vi "08 - Tip - Achieving Deterministic Handling Order.vi"() -> ()   [LabVIEW 2012]
panel:
  in  "Generate Events":enum16{"Greater than 1msec", "Sub-millisecond"}(ring)
  in  "Control":bool
  out "Static Event Registration":i32(graph)
  out "Dynamic Event Registration":i32(graph)
  out "Unique Event Queue":i32(graph)
  # "Conclusion:\nAll events within a single Events Queue will be handled deterministically;\nevents in separate Events Queues will be handled with approximately millisecond\naccuracy, but could become out of order with sub-millisecond resolution.\n\nNever expect deterministic handling order between separate event registrations,\nbut especially near and below 1msec threshold."
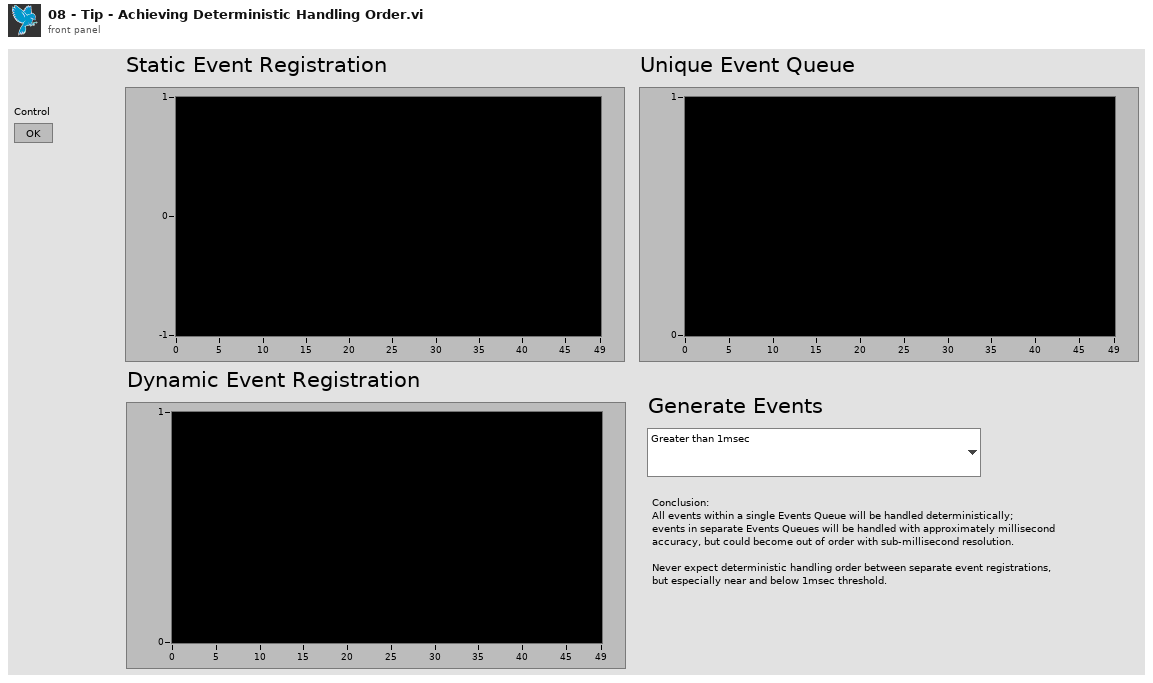
[diagram p1: front panel]
types:
  T1 = cluster{"Event Registration Refnum":refnum<event-registration>, "Event Registration Refnum":refnum<event-registration>}
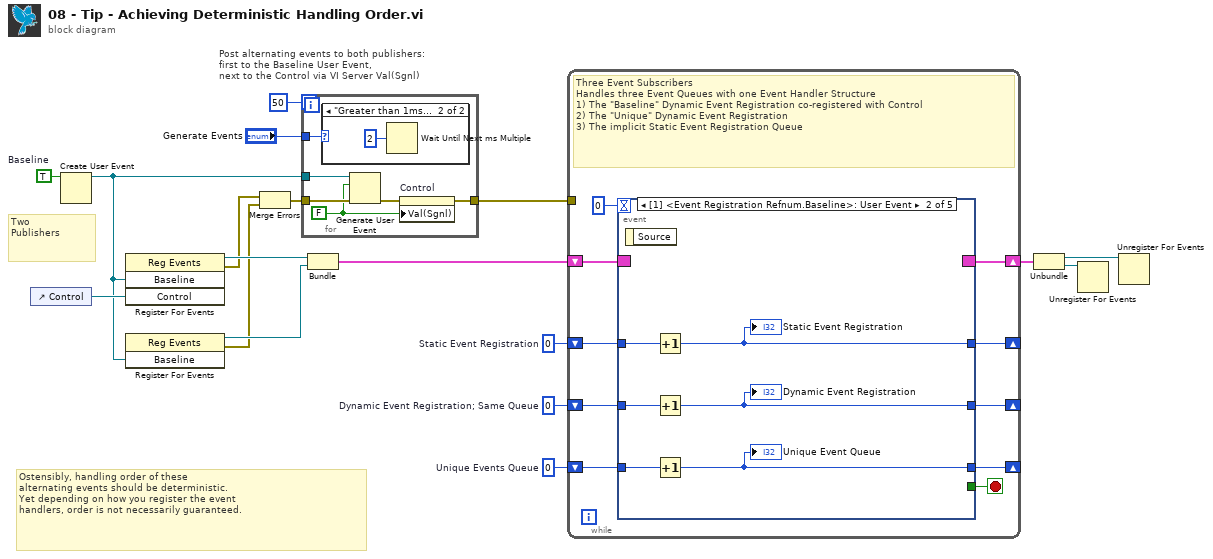
[diagram p0: block diagram]
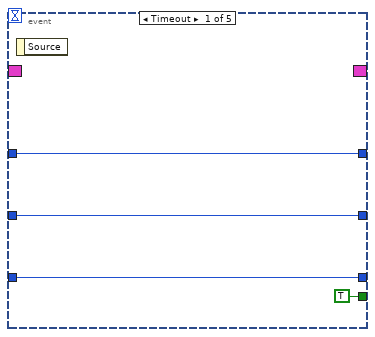
[diagram p3: hidden frame]
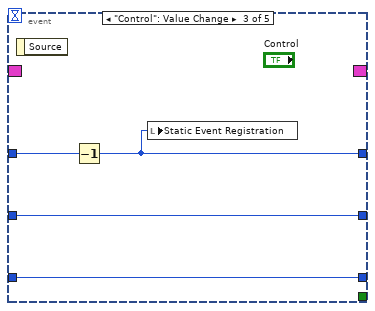
[diagram p4: hidden frame]
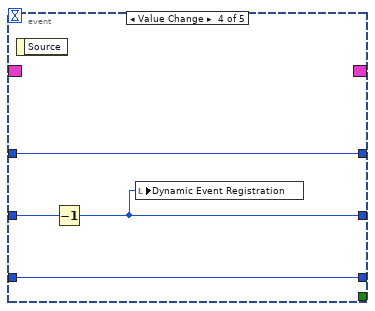
[diagram p5: hidden frame]
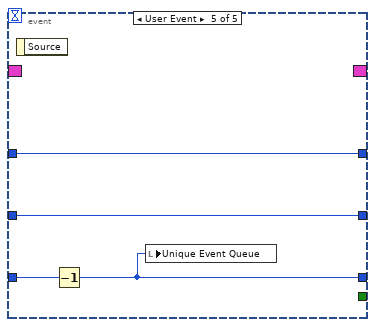
[diagram p6: hidden frame]
diagram:
  w8 = 0  # Unique Events Queue
  w13 = 0  # Dynamic Event Registration; Same Queue
  w15 = 0  # Static Event Registration
  w18 = TRUE  # Baseline
  # "Two\nPublishers"
  # "Ostensibly, handling order of these\nalternating events should be deterministic.\nYet depending on how you register the event\nhandlers, order is not necessarily guaranteed."
  n1 = control-ref of="Control"() -> (w14:refnum<vi>)
  n2 = Create User Event(user event datatype=w18) -> (user event=w12:refnum<user-event>)  [unwired: 1 in, 1 out]
  n3 = register-events(w12, w14) -> (reference out=w11:refnum<event-registration>, error out=w7:errorcluster)  [unwired: 2 in]
  n4 = register-events(w12) -> (reference out=w9:refnum<event-registration>, error out=w6:errorcluster)  [unwired: 2 in]
  n5 = Merge Errors(w7, w6) -> (w5:errorcluster)
  n6 = for "Post alternating events to both publishers:\nfirst to the Baseline User Event,\nnext to the Control via VI Server Val(Sgnl)" {
    N: 50 -> [_]
    tunnel: w12 -> [w23]
    tunnel: w5 -> [w22]
    tunnel: [w21] -> w16
    tunnel: "Generate Events" -> [w19]
    w20 = FALSE ("Value (Signaling)")
    n7 = case shown="\"Greater than 1msec\"" w19 {
      frame "Sub-millisecond" {
      }
      frame "Greater than 1msec" {
        n8 = Wait Until Next ms Multiple(millisecond multiple=u32 2 ("milliseconds to wait")) -> ()  [unwired: 1 out]
      }
    }
    n9 = Generate User Event(user event=w23, event data cluster=w20, error in=w22) -> (error out=w24:errorcluster)  [unwired: 1 out]
    n10 = property on="Control" class="Bool (strict)"(error in=w24, "Val(Sgnl)"=w20) -> (error out=w21:errorcluster)  [unwired: 1 in, 1 out]
  }
  n11 = Bundle("Event Registration Refnum"=w11, "Event Registration Refnum"=w9) -> (w10:T1)  [unwired: 1 in]
  n12 = while {
    tunnel: w16 -> [_]
    shift-right: [w31] -> _
    shift-left: w15 -> [w32]
    shift-right: [w29] -> _
    shift-left: w13 -> [w30]
    shift-right: [w28] -> _
    shift-left: w8 -> [w27]
    shift-right: [w26] -> w3
    shift-left: w10 -> [w35]
    stop <- w34 stop-if-true
    # "Three Event Subscribers\nHandles three Event Queues with one Event Handler Structure\n1) The \"Baseline\" Dynamic Event Registration co-registered with Control\n2) The \"Unique\" Dynamic Event Registration\n3) The implicit Static Event Registration Queue"
    n13 = event shown="[1] <Event Registration Refnum.Baseline>: User Event" {
      selector: w35 -> [_ _ _ _ _]
      dyn-events: [_ _ _ _ _] -> w26
      timeout: 0 -> [_ _ _ _ _]
      tunnel: [TRUE _ _ _ _] -> w34
      tunnel: w32 -> [w38 w45 w49 w52 w57]
      tunnel: [w38 w40 w46 w52 w57] -> w31
      tunnel: w30 -> [w37 w44 w48 w53 w55]
      tunnel: [w37 w41 w48 w50 w55] -> w29
      tunnel: [w36 w42 w47 w51 w54] -> w28
      tunnel: w27 -> [w36 w43 w47 w51 w56]
      event Timeout {
        n14 = event-data() -> ()  [unwired: 1 in, 1 out]
      }
      event User Event {
        n15 = event-data() -> ()  [unwired: 1 in, 1 out]
        n16 = Increment(x=w45) -> (x+1=w40:i32)
        "Static Event Registration" <- w40
        n17 = Increment(x=w44) -> (x+1=w41:i32)
        "Dynamic Event Registration" <- w41
        n18 = Increment(x=w43) -> (x+1=w42:i32)
        "Unique Event Queue" <- w42
      }
      event "Control": Value Change {
        n19 = event-data() -> ()  [unwired: 1 in, 1 out]
        n20 = Decrement(x=w49) -> (x-1=w46:i32)
        n21 = local write "Static Event Registration"(w46) -> ()
      }
      event Value Change {
        n22 = event-data() -> ()  [unwired: 1 in, 1 out]
        n23 = Decrement(x=w53) -> (x-1=w50:i32)
        n24 = local write "Dynamic Event Registration"(w50) -> ()
      }
      event User Event {
        n25 = event-data() -> ()  [unwired: 1 in, 1 out]
        n26 = Decrement(x=w56) -> (x-1=w54:i32)
        n27 = local write "Unique Event Queue"(w54) -> ()
      }
    }
  }
  n28 = Unbundle(w3) -> ("Event Registration Refnum"=w1:refnum<event-registration>, "Event Registration Refnum"=w2:refnum<event-registration>)
  n29 = Unregister For Events(event registration refnum=w2) -> ()  [unwired: 1 in, 1 out]
  n30 = Unregister For Events(event registration refnum=w1) -> ()  [unwired: 1 in, 1 out]
